vi "OE1022D Example All Data.vi"() -> ()   [LabVIEW 2022 SP3]
uses:
  C:/Users/Public/OneDrive/Desktop/PMT program/SampleCodeLabView/Kinesis_with_LabVIEW_Examples_LV12 - v3/Thorlabs.MotionControl.Controls.dll
  PMT program/SampleCodeLabView/Kinesis_with_LabVIEW_Examples_LV12 - v3/Thorlabs.MotionControl.Controls.dll
  C:/Users/Public/OneDrive/Desktop/PMT program/SampleCodeLabView/Kinesis_with_LabVIEW_Examples_LV12 - v3/Thorlabs.MotionControl.Benchtop.StepperMotorCLI.dll
  PMT program/SampleCodeLabView/Kinesis_with_LabVIEW_Examples_LV12 - v3/Thorlabs.MotionControl.Benchtop.StepperMotorCLI.dll
  <vilib>/Utility/file.llb/Write Delimited Spreadsheet (string).vi
  <vilib>/Utility/file.llb/Write Delimited Spreadsheet (DBL).vi
  C:/Users/Public/OneDrive/Desktop/PMT program/SampleCodeLabView/Kinesis_with_LabVIEW_Examples_LV12 - v3/Thorlabs.MotionControl.GenericMotorCLI.dll
  PMT program/SampleCodeLabView/Kinesis_with_LabVIEW_Examples_LV12 - v3/Thorlabs.MotionControl.GenericMotorCLI.dll
panel:
  in  "Boolean":bool
  out "Waveform Chart 2":dbl[](graph)
  out "Waveform Chart":dbl[](graph)
  out "Waveform Graph 2":dbl[](graph)
  out "Waveform Graph":dbl[](graph)
  in  "SPD":dbl=75.0 caption="Start Position\nRead Data"
  out "Steps Total":i32=67 caption="Total Steps"
  in  "Range":i32=10 caption="Range(mm)"
  in  "Header":string
  in  "file path (dialog if empty) 2":path=path "C:/Users/Public/OneDrive/Desktop/reflectivity/roughrunMOte2_2.txt"
  out "PC":dbl=750.219921875 caption="Current \nPosition" format="%#_6f"
  in  "SSD":dbl=0.15 caption="Step Size\nRead Data" format="%.4g"
  in  "WT":i32=500 caption="Wait Time (ms)\n Set Data"
  in  "Motor Controller\nSerialNumber":string="40837323"
  in  "BenchtopStepperControl":refnum<k24>(container)
  out "θh1 (°) 2":sgl caption="θh1 (deg)" format="%.2f"
  out "Rh1 2":sgl caption="Rh1 (Vrms)" format="%.3p"
  out "Yh1 2":sgl caption="Yh1 (Vrms)" format="%.3p"
  out "Xh1 2":sgl caption="Xh1 (Vrms)" format="%.3p"
  out "Xh2 2":sgl caption="Xh2 (Vrms)" format="%.3p"
  out "Yh2 2":sgl caption="Yh2 (Vrms)" format="%.3p"
  out "Rh2 2":sgl caption="Rh2 (Vrms)" format="%.3p"
  out "噪声 2":sgl caption="Noise(Vrms)" format="%.3p"
  out "频率 (Hz) 2":sgl caption="Freq (Hz)" format="%#.3f"
  out "θ (°) 2":sgl caption="θ (deg)" format="%.2f"
  out "R 2":sgl caption="R (Vrms)" format="%.3p"
  out "Y 2":sgl caption="Y (Vrms)" format="%.3p"
  out "θh2 (°) 2":sgl caption="θh2 (deg)" format="%.2f"
  out "X 2":sgl caption="X (Vrms)" format="%.3p"
  out "Yh1":sgl caption="Yh1 (Vrms)" format="%.3p"
  out "Xh1":sgl caption="Xh1 (Vrms)" format="%.3p"
  out "θh2 (°)":sgl caption="θh2 (deg)" format="%.2f"
  out "Yh2":sgl caption="Yh2 (Vrms)" format="%.3p"
  out "Xh2":sgl caption="Xh2 (Vrms)" format="%.3p"
  out "Rh2":sgl caption="Rh2 (Vrms)" format="%.3p"
  out "θh1 (°)":sgl caption="θh1 (deg)" format="%.2f"
  out "Rh1":sgl caption="Rh1 (Vrms)" format="%.3p"
  out "噪声":sgl caption="Noise(Vrms)" format="%.3p"
  out "频率 (Hz)":sgl caption="Freq (Hz)" format="%#.3f"
  out "θ (°)":sgl caption="θ (deg)" format="%.2f"
  out "Y":sgl caption="Y (Vrms)" format="%.3p"
  out "X":sgl caption="X (Vrms)" format="%.3p"
  out "R":sgl caption="R (Vrms)" format="%.3p"
  out "AUX-ADC2 (V)":sgl format="%.3f"
  out "AUX-ADC1 (V)":sgl format="%.3f"
  out "AUX-ADC3 (V)":sgl format="%.3f"
  out "AUX-ADC4 (V)":sgl format="%.3f"
  out "错误输出":errorcluster
  out "序列号":string
  in  "OE1022D":refnum<visa-resource-name>
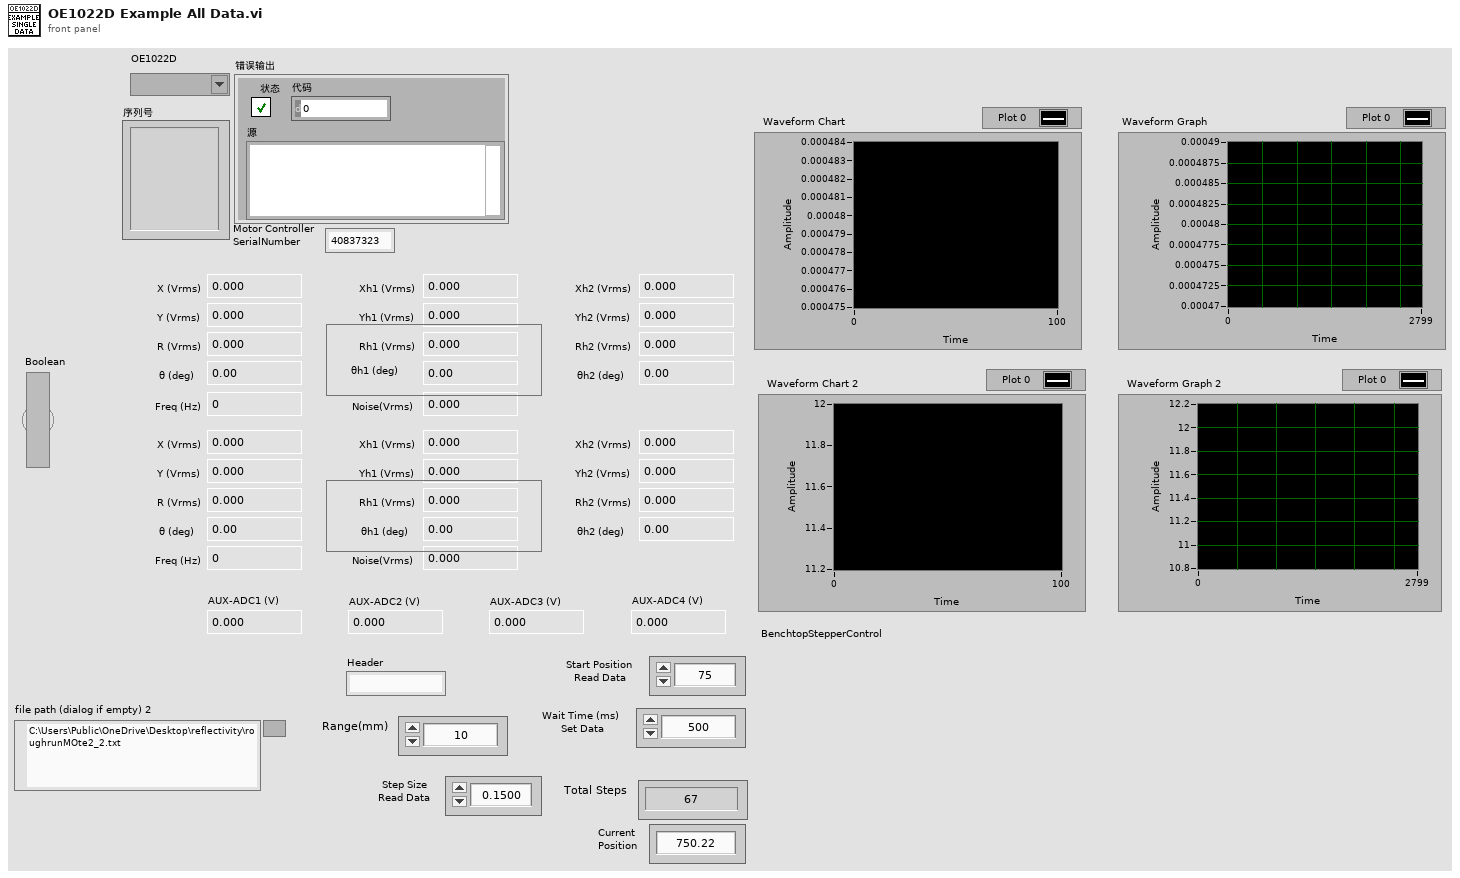
[diagram p1: front panel]
types:
  T1 = cluster{"AD1":dbl[], "AD2":dbl[], "AD3":dbl[], "AD4":dbl[]}
  T2 = cluster{"XB":dbl[], "YB":dbl[], "FrequencyB":dbl[], "NoiseB":dbl[], "Xh1B":dbl[], "Yh1B":dbl[], "Xh2B":dbl[], "Yh2B":dbl[], "Xh2B":dbl[]}
  T3 = cluster{"XA":dbl[], "YA":dbl[], "FrequencyA":dbl[], "NoiseA":dbl[], "Xh1A":dbl[], "Yh1A":dbl[], "Xh2A":dbl[], "Yh2A":dbl[]}
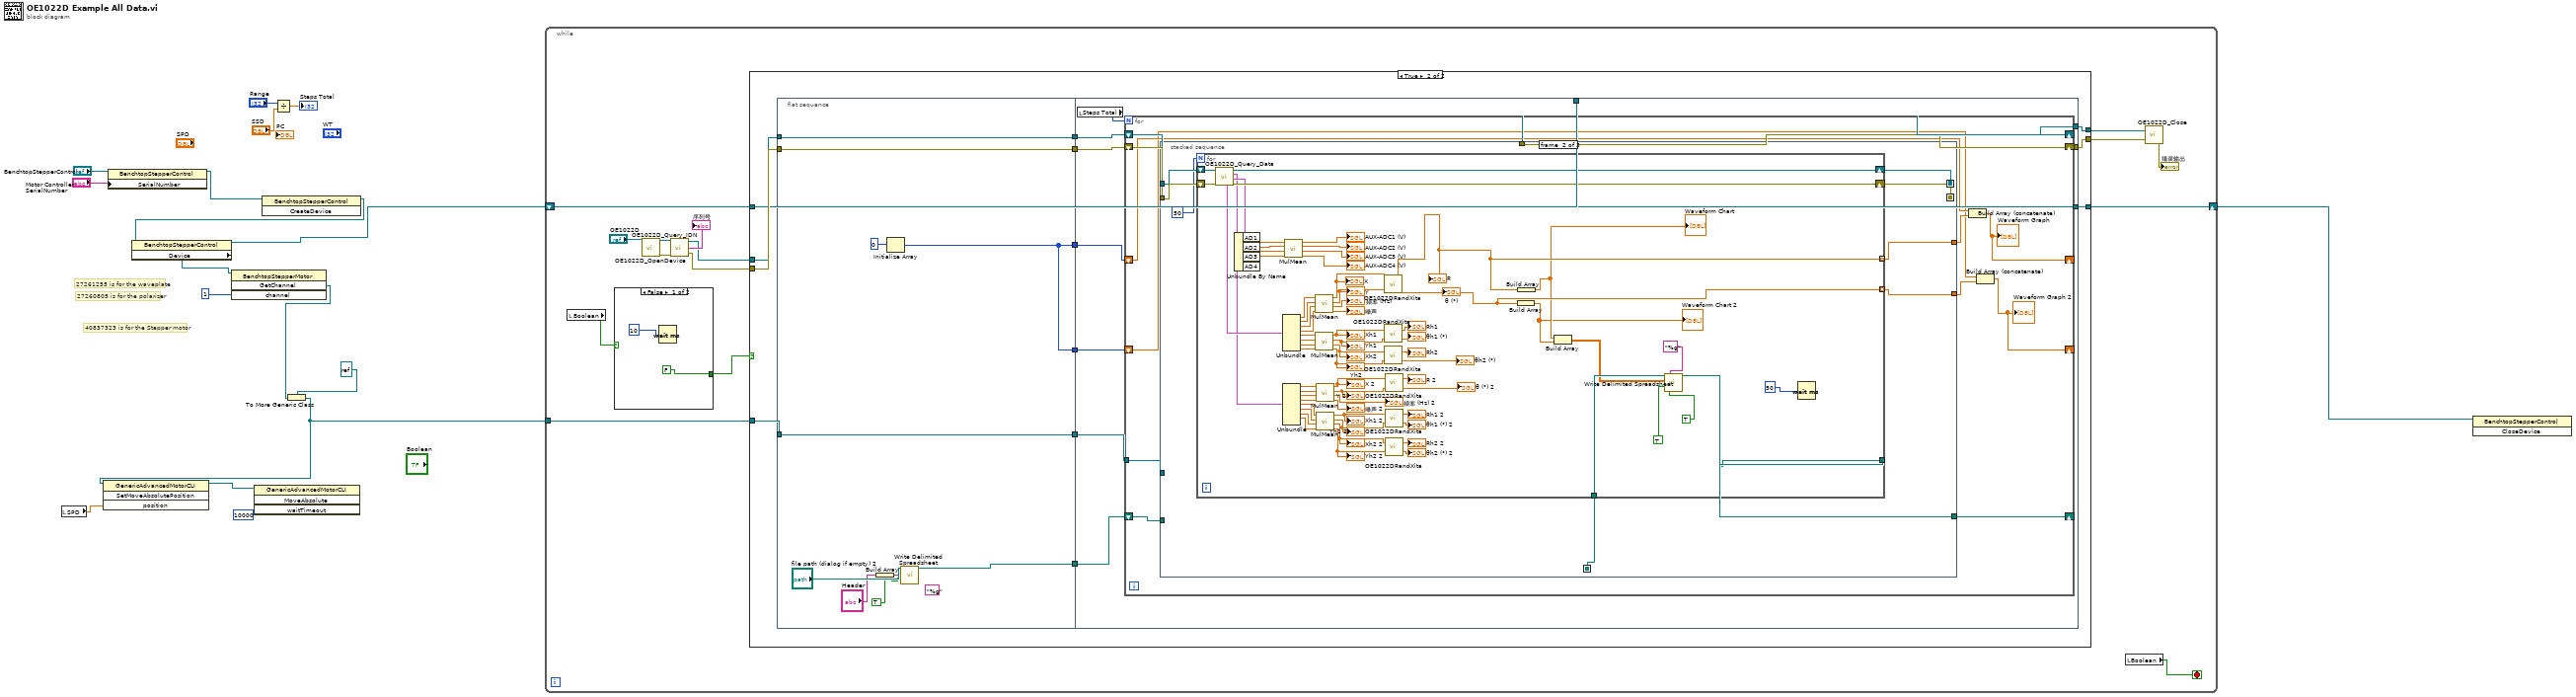
[diagram p0: block diagram]
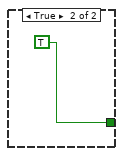
[diagram p2: hidden frame]
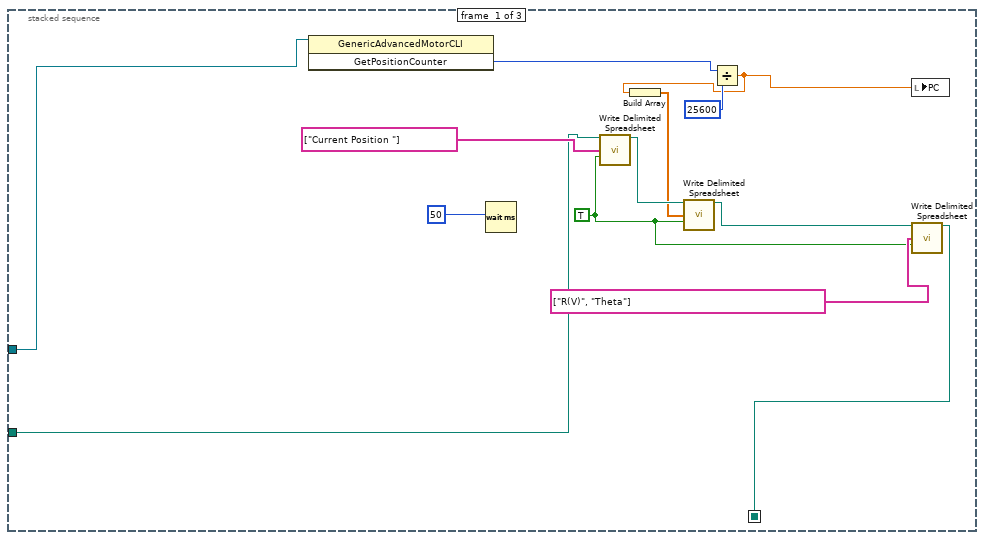
[diagram p4: hidden frame]
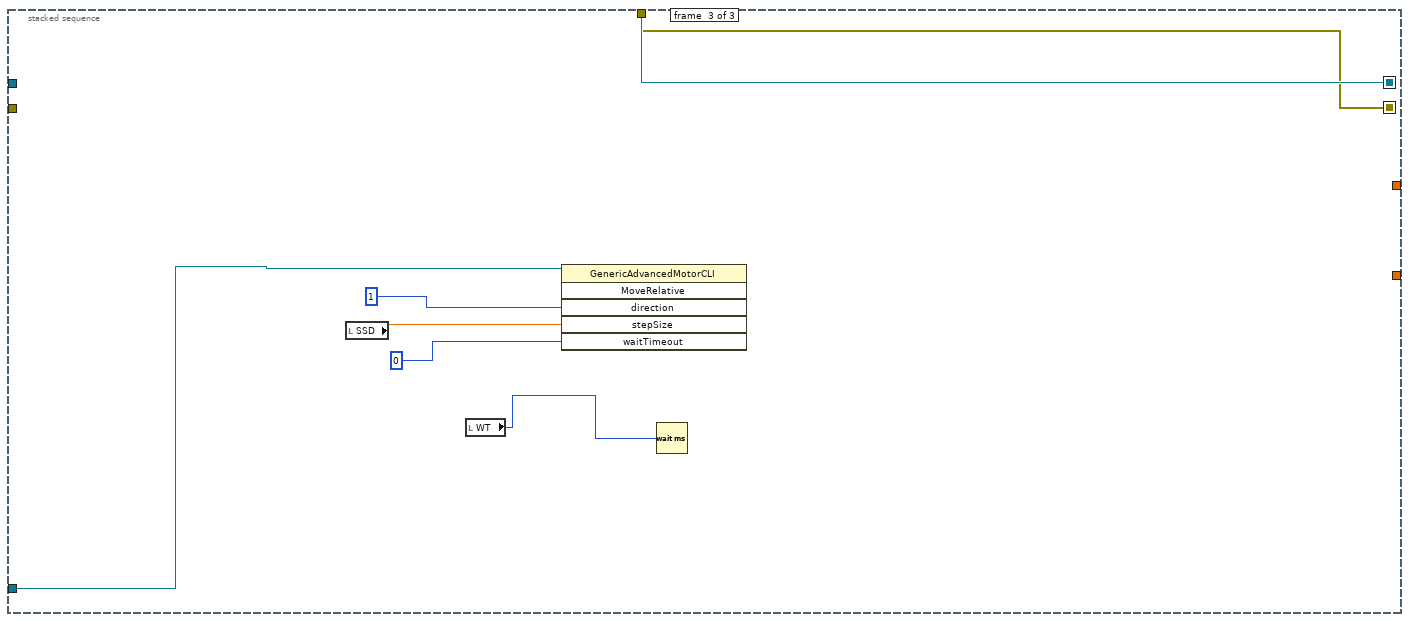
[diagram p5: hidden frame]
diagram:
  # "40837323 is for the Stepper motor"
  # "27260805 is for the polarizer"
  # "27261255 is for the waveplate"
  n1 = local read "SPD"() -> (w7:dbl)
  n2 = property class="BenchtopStepperControl"(reference="BenchtopStepperControl", "SerialNumber"="Motor Controller\nSerialNumber") -> (reference out=w11:refnum<k24>)  [unwired: 1 in, 1 out]
  n3 = invoke class="BenchtopStepperControl" method="CreateDevice"(reference=w11) -> (reference out=w1:refnum<k24>)  [unwired: 2 in, 2 out]
  n4 = property class="BenchtopStepperControl"(reference=w1) -> (reference out=w2:refnum<k24>, "Device"=w10:refnum<k24>)  [unwired: 1 in, 1 out]
  n5 = invoke class="BenchtopStepperMotor" method="GetChannel"(reference=w10, "channel"=1) -> ("GetChannel"=w9:refnum<k24>)  [unwired: 2 in, 3 out]
  n6 = Divide(x="Range", y="SSD") -> (x/y=→"Steps Total":dbl)
  n7 = To More Generic Class(target class=refnum<k24> refnum, reference=w9) -> (generic class reference=w3:refnum<k24>)
  n8 = invoke class="GenericAdvancedMotorCLI" method="SetMoveAbsolutePosition"(reference=w3, "position"=w7) -> (reference out=w8:refnum<k24>)  [unwired: 2 in, 3 out]
  n9 = invoke class="GenericAdvancedMotorCLI" method="MoveAbsolute"(reference=w8, "waitTimeout"=10000) -> ()  [unwired: 2 in, 4 out]
  n10 = while {
    tunnel: w3 -> [w25]
    shift-right: [w26] -> w14
    shift-left: w2 -> [w24]
    stop <- w19 stop-if-true
    n11 = local read "Boolean"() -> (w18:bool)
    n12 = case shown="False" w18 {
      tunnel: [FALSE TRUE] -> w20
      frame False {
        n13 = Wait (ms)(milliseconds to wait=10) -> ()  [unwired: 1 out]
      }
      frame True {
      }
    }
    n14 = call "OE1022D_OpenDevice.vi"("VISA resource name"="OE1022D") -> ("VISA资源名称输出"=w29:refnum<visa-resource-name>, "错误输出"=w31:errorcluster)  [unwired: 17 in]
    n15 = call "OE1022D_Query_IDN.vi"("错误输入（无错误）"=w31, "VISA resource name"=w29) -> ("错误输出"=w28:errorcluster, "序列号"=→"序列号":string, "VISA resource name out"=w27:refnum<visa-resource-name>)  [unwired: 1 in]
    n16 = case shown="True" w20 {
      tunnel: w28 -> [w36 w47]
      tunnel: w27 -> [w37 w46]
      tunnel: [w38 w45] -> w26
      tunnel: w25 -> [_ w44]
      tunnel: w24 -> [w38 w43]
      tunnel: [w36 w42] -> w22
      tunnel: [w37 w41] -> w21
      frame False {
      }
      frame True {
        n17 = flat-sequence {
          tunnel: [w56] -> w51
          tunnel: [w55] -> w50
          tunnel: [w54] -> w49
          tunnel: [w58] -> w48
          tunnel: w47 -> [w56]
          tunnel: w46 -> [w55]
          tunnel: w44 -> [w54]
          tunnel: [w52] -> w40
          tunnel: [w52] -> w39
          tunnel: w51 -> [w71]
          tunnel: w50 -> [w70]
          tunnel: w49 -> [w69]
          tunnel: w48 -> [w68]
          tunnel: [w67] -> w41
          tunnel: [w66] -> w42
          tunnel: [w64] -> w45
          tunnel: w43 -> [w64]
          tunnel: w40 -> [w63]
          tunnel: w39 -> [w62]
          frame #0 {
            (unwired) "%g" ("format (%.3f)")
            n18 = Build Array("Header") -> (w59:string[])
            n19 = Initialize Array(0) -> (w52:i32[])  [unwired: 1 in]
            n20 = call-poly <vilib>:"Write Delimited Spreadsheet.vi"("file path (dialog if empty)"="file path (dialog if empty) 2", "1D data"=w59, "append to file? (new file:F)"=TRUE) -> ("new file path (Not A Path if cancelled)"=w58:path)  [unwired: 11 in, 1 out]
          }
          frame #1 {
            n21 = local read "Steps Total"() -> (w65:i32)
            n22 = for {
              N: w65 -> [_]
              tunnel: w69 -> [w82]
              shift-right: [w78] -> w66
              shift-left: w71 -> [w84]
              shift-right: [w79] -> w67
              shift-left: w70 -> [w83]
              shift-right: [w81] -> _
              shift-left: w68 -> [w80]
              shift-right: [w75] -> _
              shift-left: w63 -> [w77]
              shift-right: [w73] -> _
              shift-left: w62 -> [w72]
              n23 = stacked-sequence {
                seq-local: [_ w105 _] -> [_ _ w181]
                seq-local: [_ w104 _] -> [_ _ w180]
                seq-local: [w91 _ _] -> [_ w101 _]
                tunnel: w84 -> [_ w106 _]
                tunnel: w83 -> [_ w103 _]
                tunnel: [_ _ w181] -> w79
                tunnel: [_ _ w180] -> w78
                tunnel: w82 -> [w97 _ w177]
                tunnel: [_ w100 _] -> w81
                tunnel: w80 -> [w89 _ _]
                tunnel: [_ w99 _] -> w76
                tunnel: [_ w98 _] -> w74
                frame #0 {
                  w88 = TRUE
                  n24 = invoke class="GenericAdvancedMotorCLI" method="GetPositionCounter"(reference=w97) -> ("GetPositionCounter"=w86:i32)  [unwired: 2 in, 2 out]
                  n25 = Wait (ms)(milliseconds to wait=50) -> ()  [unwired: 1 out]
                  n26 = call-poly <vilib>:"Write Delimited Spreadsheet.vi"("file path (dialog if empty)"=w89, "1D data"=string[] ["Current Position "], "append to file? (new file:F)"=w88) -> ("new file path (Not A Path if cancelled)"=w94:path)  [unwired: 11 in, 1 out]
                  n27 = Divide(x=w86, y=25600) -> (x/y=w85:dbl)
                  n28 = Build Array(w85) -> (w93:dbl[])
                  n29 = call-poly <vilib>:"Write Delimited Spreadsheet.vi"("file path (dialog if empty)"=w94, "1D data"=w93, "append to file? (new file:F)"=w88) -> ("new file path (Not A Path if cancelled)"=w92:path)  [unwired: 11 in, 1 out]
                  n30 = local write "PC"(w85) -> ()
                  n31 = call-poly <vilib>:"Write Delimited Spreadsheet.vi"("file path (dialog if empty)"=w92, "1D data"=string[] ["R(V)", "Theta"], "append to file? (new file:F)"=w88) -> ("new file path (Not A Path if cancelled)"=w91:path)  [unwired: 11 in, 1 out]
                }
                frame #1 {
                  n32 = for {
                    N: 50 -> [_]
                    shift-right: [w172] -> w104
                    shift-left: w106 -> [w174]
                    shift-right: [w173] -> w105
                    shift-left: w103 -> [w171]
                    tunnel: w101 -> [w170]
                    tunnel: [w169] -> w100
                    tunnel: [w111] -> w99 mode=indexing
                    tunnel: [w110] -> w98 mode=indexing
                    n33 = call "OE1022D_Query_Data.vi"("错误输入（无错误）"=w174, "VISA resource name"=w171) -> ("error out"=w172:errorcluster, "输出簇ADC"=w117:T1, "输出簇B"=w116:T2, "VISA resource name out"=w173:refnum<visa-resource-name>, "输出簇A"=w118:T3)  [unwired: 3 in]
                    n34 = Unbundle By Name(w117) -> ("AD1"=w161:dbl[], "AD2"=w162:dbl[], "AD3"=w163:dbl[], "AD4"=w164:dbl[])
                    n35 = Unbundle(w118) -> ("XA"=w123:dbl[], "YA"=w124:dbl[], "FrequencyA"=w125:dbl[], "NoiseA"=w126:dbl[], "Xh1A"=w131:dbl[], "Yh1A"=w132:dbl[], "Xh2A"=w133:dbl[], "Yh2A"=w134:dbl[])
                    n36 = Unbundle(w116) -> ("XB"=w148:dbl[], "YB"=w147:dbl[], "FrequencyB"=w146:dbl[], "NoiseB"=w145:dbl[], "Xh1B"=w144:dbl[], "Yh1B"=w143:dbl[], "Xh2B"=w142:dbl[], "Yh2B"=w141:dbl[])  [unwired: 1 out]
                    n37 = call "MulMean.vi"("IN 4"=w164, "IN 3"=w163, "IN 2"=w162, "IN 1"=w161) -> ("mean 4"=→"AUX-ADC4 (V)":dbl, "mean 3"=→"AUX-ADC3 (V)":dbl, "mean 2"=→"AUX-ADC2 (V)":dbl, "mean 1"=→"AUX-ADC1 (V)":dbl)  [unwired: 4 in]
                    n38 = call "MulMean.vi"("IN 4"=w126, "IN 3"=w125, "IN 2"=w124, "IN 1"=w123) -> ("mean 4"=→"噪声":dbl, "mean 3"=→"频率 (Hz)":dbl, "mean 2"=w129:dbl, "mean 1"=w128:dbl)  [unwired: 4 in]
                    "X" <- w128
                    "Y" <- w129
                    n39 = call "MulMean.vi"("IN 4"=w134, "IN 3"=w133, "IN 2"=w132, "IN 1"=w131) -> ("mean 4"=w138:dbl, "mean 3"=w137:dbl, "mean 2"=w136:dbl, "mean 1"=w135:dbl)  [unwired: 4 in]
                    "Xh2" <- w137
                    "Yh2" <- w138
                    "Xh1" <- w135
                    "Yh1" <- w136
                    n40 = call "MulMean.vi"("IN 4"=w145, "IN 3"=w146, "IN 2"=w147, "IN 1"=w148) -> ("mean 4"=→"噪声 2":dbl, "mean 3"=→"频率 (Hz) 2":dbl, "mean 2"=w154:dbl, "mean 1"=w153:dbl)  [unwired: 4 in]
                    "X 2" <- w153
                    "Y 2" <- w154
                    n41 = call "MulMean.vi"("IN 4"=w141, "IN 3"=w142, "IN 2"=w143, "IN 1"=w144) -> ("mean 4"=w158:dbl, "mean 3"=w157:dbl, "mean 2"=w156:dbl, "mean 1"=w155:dbl)  [unwired: 4 in]
                    "Yh2 2" <- w158
                    "Xh2 2" <- w157
                    "Xh1 2" <- w155
                    "Yh1 2" <- w156
                    n42 = call "OE1022DRandXita.vi"("Y"=w129, "X"=w128) -> ("θ (°)"=w110:dbl, "R"=w111:dbl)
                    "R" <- w111
                    "θ (°)" <- w110
                    n43 = call "OE1022DRandXita.vi"("Y"=w136, "X"=w135) -> ("θ (°)"=→"θh1 (°)":dbl, "R"=→"Rh1":dbl)
                    n44 = call "OE1022DRandXita.vi"("Y"=w138, "X"=w137) -> ("θ (°)"=→"θh2 (°)":dbl, "R"=→"Rh2":dbl)
                    n45 = call "OE1022DRandXita.vi"("Y"=w154, "X"=w153) -> ("θ (°)"=→"θ (°) 2":dbl, "R"=→"R 2":dbl)
                    n46 = call "OE1022DRandXita.vi"("Y"=w156, "X"=w155) -> ("θ (°)"=→"θh1 (°) 2":dbl, "R"=→"Rh1 2":dbl)
                    n47 = call "OE1022DRandXita.vi"("Y"=w158, "X"=w157) -> ("θ (°)"=→"θh2 (°) 2":dbl, "R"=→"Rh2 2":dbl)
                    n48 = Build Array(w110) -> (w108:dbl[])
                    "Waveform Chart 2" <- w108
                    n49 = Build Array(w111) -> (w109:dbl[])
                    "Waveform Chart" <- w109
                    n50 = Build Array(w109, w108) -> (w165:dbl[][])
                    n51 = call-poly <vilib>:"Write Delimited Spreadsheet.vi"("file path (dialog if empty)"=w170, "format (%.3f)"="%g", "2D data"=w165, "append to file? (new file:F)"=TRUE, "transpose? (no:F)"=TRUE) -> ("new file path (Not A Path if cancelled)"=w169:path)  [unwired: 9 in, 1 out]
                    n52 = Wait (ms)(milliseconds to wait=50) -> ()  [unwired: 1 out]
                  }
                }
                frame #2 {
                  n53 = local read "SSD"() -> (w176:dbl)
                  n54 = local read "WT"() -> (w175:i32)
                  n55 = invoke class="GenericAdvancedMotorCLI" method="MoveRelative"(reference=w177, "direction"=1, "stepSize"=w176, "waitTimeout"=0) -> ()  [unwired: 2 in, 6 out]
                  n56 = Wait (ms)(milliseconds to wait=w175) -> ()  [unwired: 1 out]
                }
              }
              n57 = Build Array (concatenate)(w77, w76) -> (w75:dbl[])
              "Waveform Graph" <- w75
              n58 = Build Array (concatenate)(w72, w74) -> (w73:dbl[])
              "Waveform Graph 2" <- w73
            }
          }
        }
      }
    }
    n59 = local read "Boolean"() -> (w19:bool)
    n60 = call "OE1022D_Close.vi"("错误输入（无错误）"=w22, "VISA resource name"=w21) -> ("错误输出"=→"错误输出":errorcluster)  [unwired: 1 in]
  }
  n61 = invoke class="BenchtopStepperControl" method="CloseDevice"(reference=w14) -> ()  [unwired: 2 in, 3 out]
